vi "Practise Shared.vi"() -> ()   [LabVIEW 2014]
panel:
  out "counts 2":dbl
  in  "stop":bool
  out "counts":dbl
  # "Practice Shared"
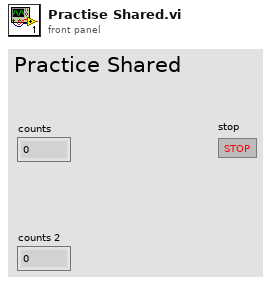
[diagram p1: front panel]
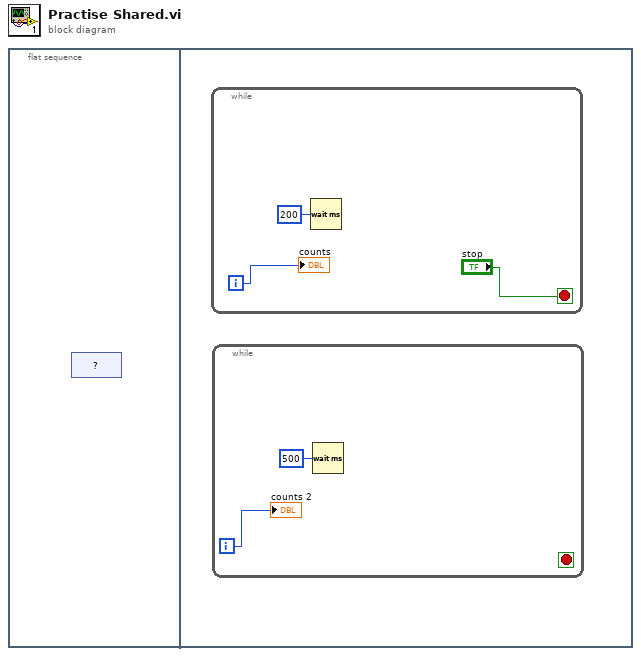
[diagram p0: block diagram]
diagram:
  n1 = flat-sequence {
    frame #0 {
      n2 = shared-variable "?"() -> ()  [unwired: 1 in, 2 out]
    }
    frame #1 {
      n3 = while {
        i -> [w5]
        stop <- "stop" stop-if-true
        n4 = Wait (ms)(milliseconds to wait=u32 200) -> ()  [unwired: 1 out]
        "counts" <- w5
      }
      n5 = while {
        i -> [w2]
        stop <- _ stop-if-true
        n6 = Wait (ms)(milliseconds to wait=u32 500) -> ()  [unwired: 1 out]
        "counts 2" <- w2
      }
    }
  }
